vi "InitializeFpgaWithTachBurstMode.vi"(8 "error in (no error)":errorcluster, 11 "923x Acquisition Config":T1={"Acq"=FALSE, "NumberOfModules"=0, "Dynamic FPGA VI Ref"=refnum, "KeyphasorX3"=[], "FixedSizeX32"={"EnabledChannels"=[], "Sensitivity"=[], "InputConfig"=[]}, "SamplingInfo"={"Number of Channels"=4, "Sampling Rate"=4.0, "Channels"=[], "Units"=[], "Offsets"=[]}, "Normal Mode Sample Rate"=0.0, "BlockSize (sec)"=0.0, "Samples To Read (per chan)"=0, "RunningAcquisitionLength"=0.0, "Settling Time"=0.0, "Fpga Tach Buffer Size (samples)"=0, "Waveform Groups"=[], "Acquisition Block Number"=0, "Device Name"="", "ValidConfig"=FALSE, "Last Dynamic Module"="", "HighPassFilterState"=[], "Low Frequency Cutoff"=[], "BurstMode"={"Acquisition Time"=0.0, "Sample Rate"=0.0, "Collection Reason"=""}} {"HighPassFilterState"."Filter State" format="%.2f"; "HighPassFilterState"."IIR Filter Cluster"."Forward Coefficients" format="%.2f"; "HighPassFilterState"."IIR Filter Cluster"."Reverse Coefficients" format="%.2f"; "FixedSizeX32"."InputConfig" items=["AC Coupled", "DC Coupled", "IEPE AC Coupled"]}) -> (0 "error out":errorcluster, 1 "start acquisition?":bool, 2 "dynamic FPGA VI reference":refnum<k20>, 3 "923x Acquisition Config out":T1={"Acq"=FALSE, "NumberOfModules"=0, "Dynamic FPGA VI Ref"=refnum, "KeyphasorX3"=[], "FixedSizeX32"={"EnabledChannels"=[], "Sensitivity"=[], "InputConfig"=[]}, "SamplingInfo"={"Number of Channels"=4, "Sampling Rate"=4.0, "Channels"=[], "Units"=[], "Offsets"=[]}, "Normal Mode Sample Rate"=0.0, "BlockSize (sec)"=0.0, "Samples To Read (per chan)"=0, "RunningAcquisitionLength"=0.0, "Settling Time"=0.0, "Fpga Tach Buffer Size (samples)"=0, "Waveform Groups"=[], "Acquisition Block Number"=0, "Device Name"="", "ValidConfig"=FALSE, "Last Dynamic Module"="", "HighPassFilterState"=[], "Low Frequency Cutoff"=[], "BurstMode"={"Acquisition Time"=0.0, "Sample Rate"=0.0, "Collection Reason"=""}} {"HighPassFilterState"."Filter State" format="%.2f"; "HighPassFilterState"."IIR Filter Cluster"."Forward Coefficients" format="%.2f"; "HighPassFilterState"."IIR Filter Cluster"."Reverse Coefficients" format="%.2f"; "FixedSizeX32"."InputConfig" items=["AC Coupled", "DC Coupled", "IEPE AC Coupled"]})   [LabVIEW 2017, in "CmsAcquisition.lvlib"]
doc: "Initializes the acquisition of the dynamic channels with the RIO Wfm API."
uses:
  <vilib>/addons/InsightCM/Devices/Shared/Cms/CmsAcquisition/CmsAcquisition.lvlib
  <vilib>/addons/InsightCM/Devices/Shared/Cms/CmsAcquisition/controls/Configuration.ctl
  <vilib>/addons/InsightCM/Devices/Shared/Cms/CmsAcquisition/controls/TachometerConfig.ctl
  <vilib>/addons/InsightCM/Devices/Shared/Cms/CmsAcquisition/controls/FixedSizeArrays.ctl
  <vilib>/LabVIEW Targets/FPGA/cRIO/shared/nicrio_ModuleControls/nicrio_cRIO-9232_ConfigModeRing.ctl
  <vilib>/addons/InsightCM/Devices/Shared/Cms/cRIOWfmAcq/subVIs/RIO Wfm Cust Ctrls/rwfm_SamplingInfo.ctl
  <vilib>/addons/InsightCM/Devices/Shared/Cms/CmsAcquisition/controls/Group.ctl
  <vilib>/addons/InsightCM/Devices/Shared/Cms/CmsAcquisition/controls/Channel.ctl
  <vilib>/addons/InsightCM/Utilities/Analysis/Vibration/controls/HighPassFilterState.ctl
  <vilib>/addons/InsightCM/Devices/Shared/Cms/CmsAcquisition/controls/BurstMode.ctl
  <vilib>/Utility/error.llb/Error Cluster From Error Code.vi
  <vilib>/rvi/errors/niLvFpgaAdjustHostInterfaceError.vi
  <vilib>/addons/InsightCM/Devices/Shared/Cms/cRIOWfmAcq/subVIs/RIO Wfm Cust Ctrls/rwfm_FPGARefTach.ctl
  <vilib>/rvi/interface/nirviReadWriteControl/nirviReadWriteControl.xnode
  <vilib>/addons/InsightCM/Devices/Shared/Cms/cRIOWfmAcq/cRIOWfmLib.lvlib
  <vilib>/rvi/interface/Simulation/niFpgaSimulationCallBeginRW.vi
  NiFpgaLv.dll
  <vilib>/addons/InsightCM/Utilities/Analysis/Vibration/VibrationAnalysisFunctions.lvlib
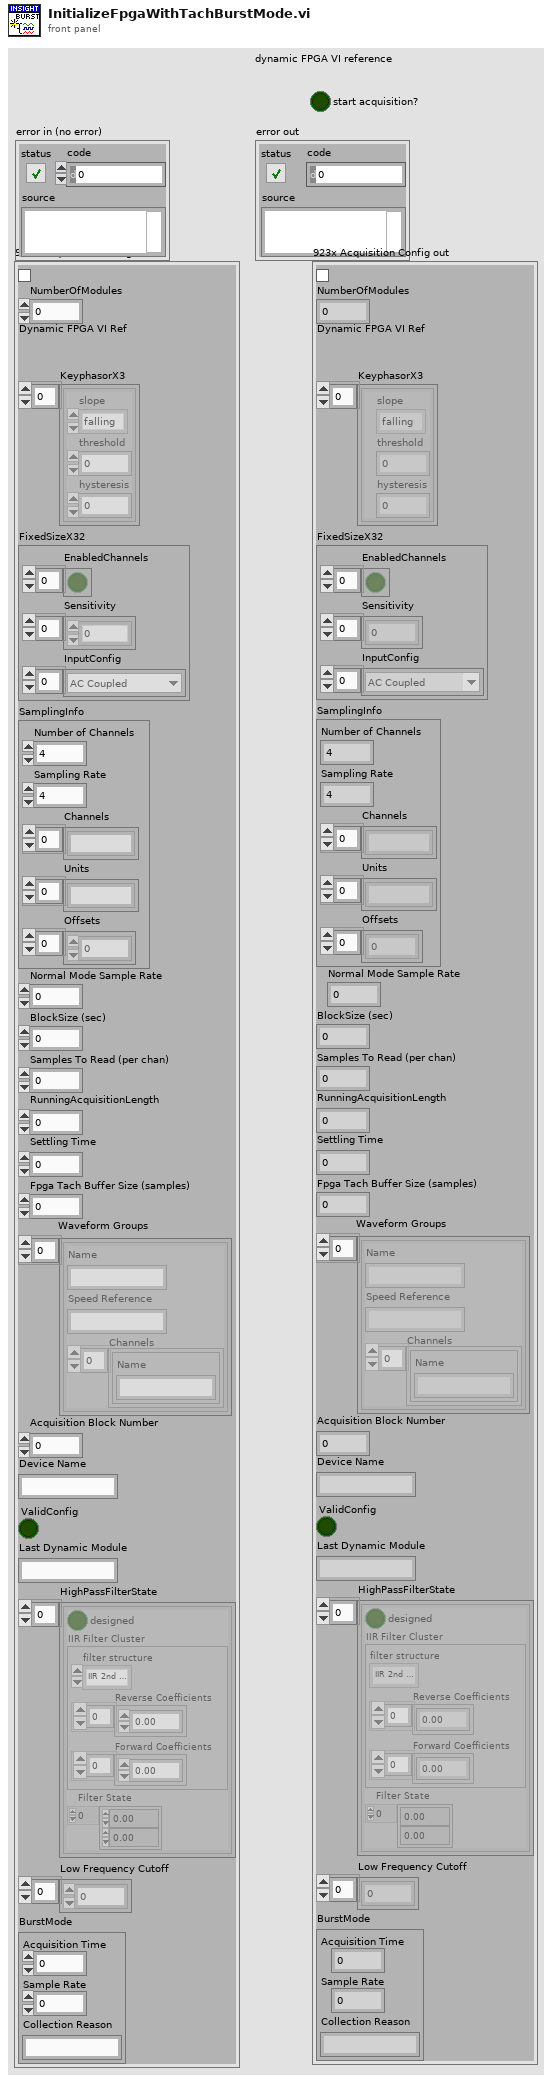
[diagram p1: front panel]
types:
  T1 = typedef "CmsAcquisition.lvlib/Configuration.ctl" = cluster{"Acq":bool, "NumberOfModules":i16, "Dynamic FPGA VI Ref":refnum<k20>, "KeyphasorX3":T2[], "FixedSizeX32":T3, "SamplingInfo":T5, "Normal Mode Sample Rate":dbl, "BlockSize (sec)":dbl, "Samples To Read (per chan)":i32, "RunningAcquisitionLength":dbl, "Settling Time":dbl, "Fpga Tach Buffer Size (samples)":i32, "Waveform Groups":T6[], "Acquisition Block Number":i32, "Device Name":string, "ValidConfig":bool, "Last Dynamic Module":string, "HighPassFilterState":T8[], "Low Frequency Cutoff":dbl[], "BurstMode":T9}
  T2 = typedef "CmsAcquisition.lvlib/TachometerConfig.ctl" = cluster{"slope":enum16{"falling", "rising"}, "threshold":dbl, "hysteresis":dbl}
  T3 = typedef "CmsAcquisition.lvlib/FixedSizeArrays.ctl" = cluster{"EnabledChannels":bool[], "Sensitivity":dbl[], "InputConfig":T4[]}
  T4 = typedef "nicrio_cRIO-9232_ConfigModeRing.ctl" = u8
  T5 = typedef "cRIOWfmLib.lvlib/rwfm_SamplingInfo.ctl" = cluster{"Number of Channels":i32, "Sampling Rate":dbl, "Channels":string[], "Units":string[], "Offsets":sgl[]}
  T6 = typedef "CmsAcquisition.lvlib/Group.ctl" = cluster{"Name":string, "Speed Reference":string, "Channels":T7[]}
  T7 = typedef "CmsAcquisition.lvlib/Channel.ctl" = cluster{"Name":string}
  T8 = typedef "VibrationAnalysisFunctions.lvlib/HighPassFilterState.ctl" = cluster{"designed":bool, "IIR Filter Cluster":cluster{"filter structure":enum32{"IIR 2nd Order", "IIR 4th Order"}, "Reverse Coefficients":dbl[], "Forward Coefficients":dbl[]}, "Filter State":dbl[]}
  T9 = typedef "CmsAcquisition.lvlib/BurstMode.ctl" = cluster{"Acquisition Time":dbl, "Sample Rate":dbl, "Collection Reason":string}
  T10 = typedef "cRIOWfmLib.lvlib/rwfm_FPGARefTach.ctl" = refnum<k20>
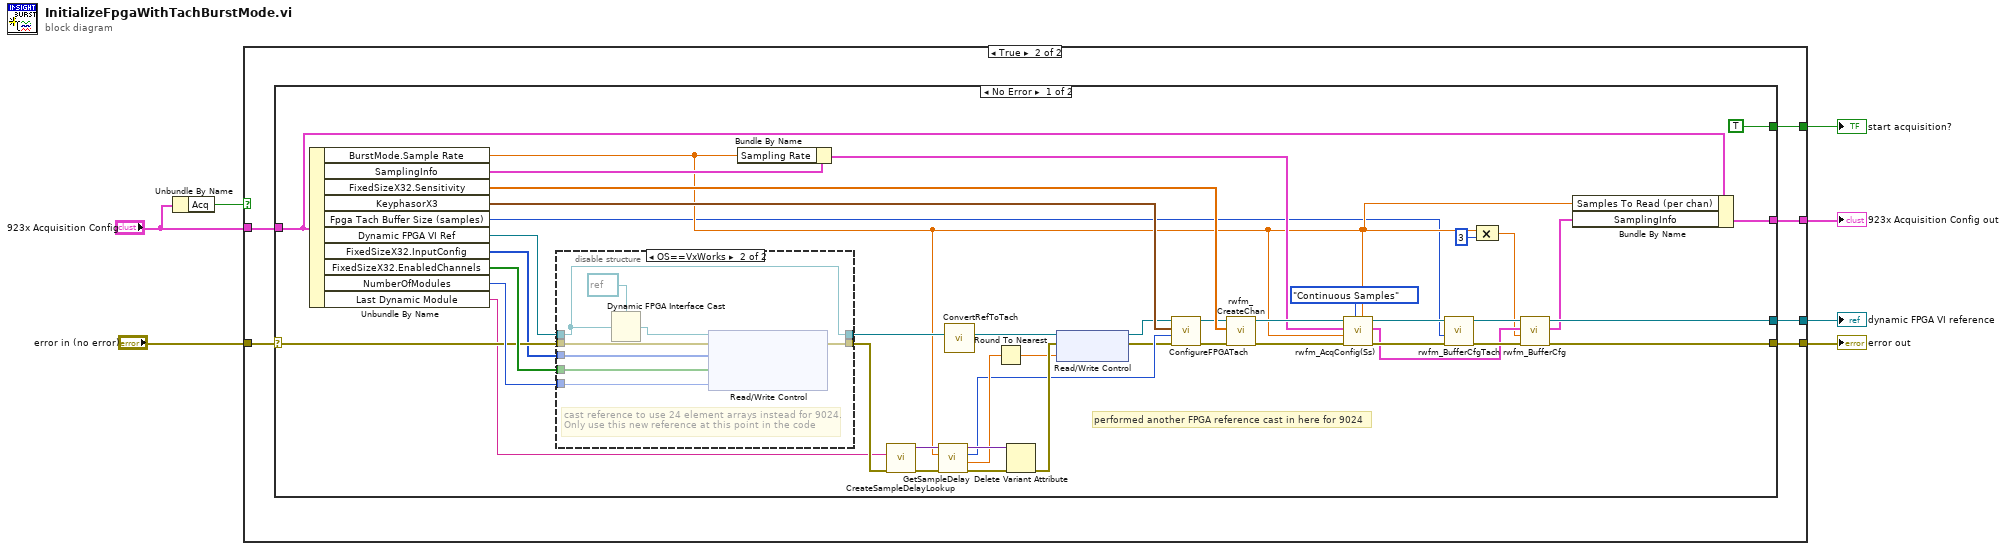
[diagram p0: block diagram]
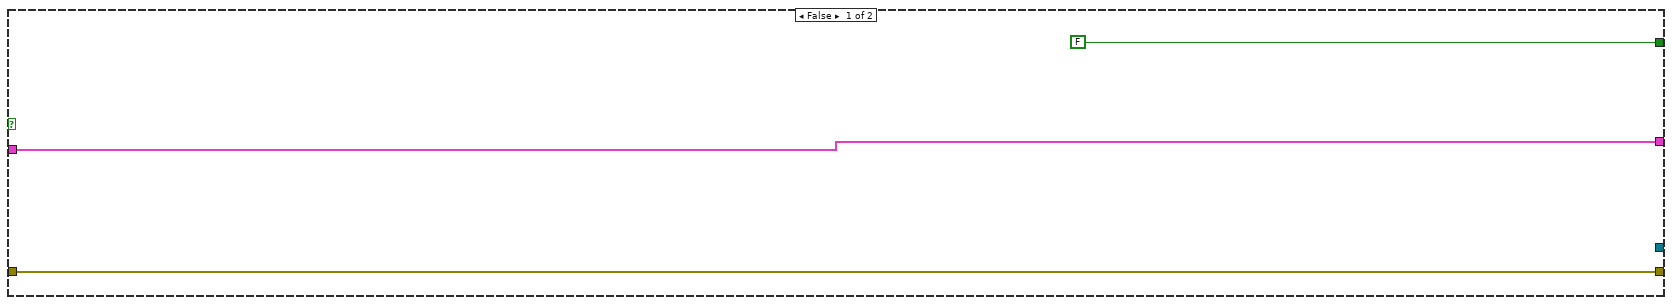
[diagram p2: hidden frame]
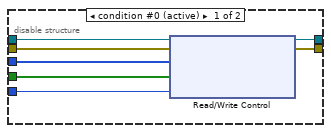
[diagram p3: hidden frame]
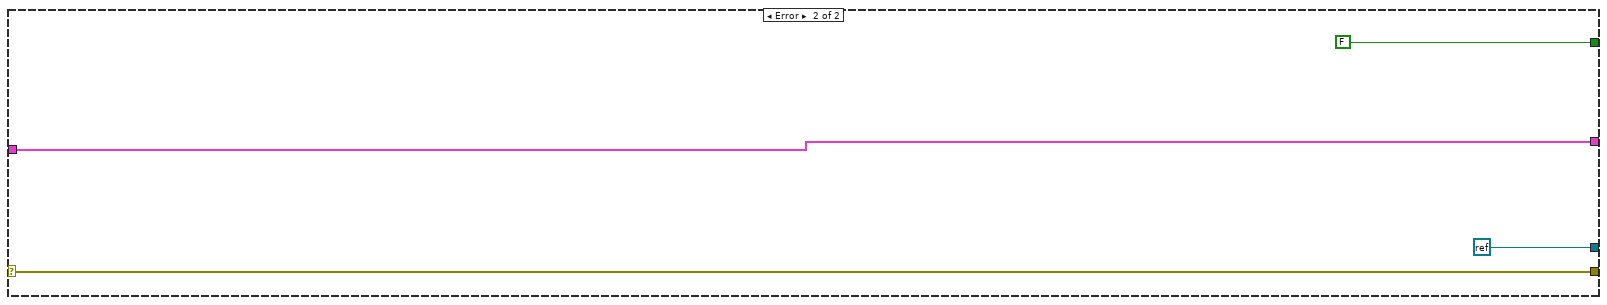
[diagram p4: hidden frame]
diagram:
  n1 = Unbundle By Name("923x Acquisition Config") -> ("Acq"=w2:bool)
  n2 = case shown="True" w2 {
    tunnel: [w10 w16] -> w7
    tunnel: "error in (no error)" -> [w10 w15]
    tunnel: [_ w14] -> w5
    tunnel: "923x Acquisition Config" -> [w8 w13]
    tunnel: [FALSE w12] -> w3
    tunnel: [w8 w11] -> w1
    frame False {
    }
    frame True {
      n3 = case shown="No Error" w15 {
        selector: w15 -> [w43 w78]
        tunnel: w13 -> [w22 w75]
        tunnel: [w25 w78] -> w16
        tunnel: [w27 refnum<k0> refnum] -> w14
        tunnel: [TRUE FALSE] -> w12
        tunnel: [w20 w75] -> w11
        frame No Error {
          # "performed another FPGA reference cast in here for 9024"
          n4 = Unbundle By Name(w22) -> ("BurstMode.Sample Rate"=w18:dbl, "SamplingInfo"=w32:T5, "FixedSizeX32.Sensitivity"=w58:dbl[], "KeyphasorX3"=w57:T2[], "Fpga Tach Buffer Size (samples)"=w17:i32, "Dynamic FPGA VI Ref"=w35:refnum<k20>, "FixedSizeX32.InputConfig"=w36:T4[], "FixedSizeX32.EnabledChannels"=w59:bool[], "NumberOfModules"=w56:i16, "Last Dynamic Module"=w33:string)
          n5 = disable-structure shown="OS==VxWorks" {
            disable-tunnel: w59 -> [w66 w68]
            disable-tunnel: w56 -> [w65 w74]
            disable-tunnel: [w64 w73] -> w48
            disable-tunnel: w43 -> [w63 w72]
            disable-tunnel: [w62 w67] -> w42
            disable-tunnel: w36 -> [w61 w69]
            disable-tunnel: w35 -> [w60 w67]
            frame condition #0 (active) {
              n6 = xnode "Read/Write Control"("FPGA VI Reference In"=w60, "error in"=w63, "Input Config Array"=w61, "Enable Chan Array"=w66, "Number of Modules"=w65) -> ("FPGA VI Reference Out"=w62:refnum<k20>, "error out"=w64:errorcluster)
            }
            frame condition #1 {
              # "cast reference to use 24 element arrays instead for 9024.\nOnly use this new reference at this point in the code"
              n7 = Dynamic FPGA Interface Cast(Session In=refnum<k20> refnum ("FPGA VI Reference In"), Type=w67) -> (Session Out=w70:refnum<k20>)
              n8 = xnode "Read/Write Control"("FPGA VI Reference In"=w70, "error in"=w72, "Input Config Array"=w69, "Enable Chan Array"=w68, "Number of Modules"=w74) -> ("error out"=w73:errorcluster)  [unwired: 1 out]
            }
          }
          n9 = Bundle By Name(cluster=w32, "Sampling Rate"=w18) -> (w31:T5)
          n10 = call <vilib>:"CreateSampleDelayLookup.vi"("error in"=w48, "Last Dynamic Module"=w33) -> ("error out"=w49:errorcluster, "lookup"=w52:variant)  [unwired: 8 in]
          n11 = call <vilib>:"GetSampleDelay.vi"("error in (no error)"=w49, "sample rate"=w18, "lookup"=w52) -> ("error out"=w51:errorcluster, "delay compensation (samples)"=w47:dbl, "delay compensation (OS clocks)"=w45:u32, "lookup"=w50:variant)  [unwired: 5 in]
          n12 = call <vilib>:"ConvertRefToTach.vi"("FPGA Ref"=w42) -> ("FPGA Ref"=w41:T10)  [unwired: 10 in]
          n13 = Round To Nearest(number=w47) -> (nearest integer value=w44:dbl)
          n14 = Delete Variant Attribute(4:w51, 7:w50) -> (0:w46:errorcluster)  [unwired: 1 in, 2 out]
          n15 = xnode "Read/Write Control"("FPGA VI Reference In"=w41, "error in"=w46, "Tach Delay"=w44) -> ("FPGA VI Reference Out"=w37:T10, "error out"=w40:errorcluster)
          n16 = call <vilib>:"ConfigureFPGATach.vi"("error in (no error)"=w40, "delay comp"=w45, "keyphasor config"=w57, "dynamic FPGA VI reference"=w37) -> ("error out"=w53:errorcluster, "dynamic FPGA VI reference"=w38:T10)  [unwired: 6 in]
          n17 = call <vilib>:"rwfm_CreateChan.vi"("error in"=w53, "Sensitivity"=w58, "Dynamic FPGA VI Reference"=w38) -> ("error out"=w54:errorcluster, "Dynamic FPGA VI Reference"=w39:T10)  [unwired: 7 in]
          n18 = call <vilib>:"rwfm_AcqConfig(Ss).vi"("Samples per Channel"=w18, "Sample Mode"=enum16{"Finite Samples", "Continuous Samples"}."Continuous Samples", "error in"=w54, "Sample Rate S/s"=w18, "Sampling Info In"=w31, "Dynamic FPGA Ref"=w39) -> ("error out"=w29:errorcluster, "Sampling Info Out"=w24:T5, "Dynamic FPGA Ref Out"=w30:T10)  [unwired: 2 in, 1 out]
          n19 = call <vilib>:"rwfm_BufferCfgTach.vi"("error in"=w29, "Buffer Size [Total Samples]"=w17, "Dynamic FPGA VI Reference"=w30) -> ("error out"=w26:errorcluster, "FPGA VI Reference Out"=w28:T10)  [unwired: 6 in, 1 out]
          n20 = Compound Arithmetic op=MULTIPLY(w18, 3 ("value")) -> (w19:dbl)
          n21 = call <vilib>:"rwfm_BufferCfg.vi"("error in"=w26, "Buffer Size [Samps per Chan]"=w19, "Sampling Info In"=w24, "Dynamic FPGA VI Reference"=w28) -> ("error out"=w25:errorcluster, "Sampling Info Out"=w21:T5, "Dynamic FPGA VI Reference"=w27:T10)  [unwired: 4 in, 1 out]
          n22 = Bundle By Name(cluster=w22, "Samples To Read (per chan)"=w18, "SamplingInfo"=w21) -> (w20:T1)
        }
        frame Error {
        }
      }
    }
  }
  "error out" <- w7
  "dynamic FPGA VI reference" <- w5
  "start acquisition?" <- w3
  "923x Acquisition Config out" <- w1
